vi "Create Suspected Pixels List.vi"(6 "IP Results":T1, 9 "tolerance":i32, 10 "Y Points":i16[](array[numeric]), 11 "X Points":i16[](array[numeric])) -> (1 "SuspPixelsIndex":u32[](array[numeric]), 2 "SuspPixelsY":u32[](array[numeric]), 3 "SuspPixelsX":u32[](array[numeric]))   [LabVIEW 2015]
uses:
  IP results.ctl
panel:
  out "Intensity Graph":u8[][](graph)
  out "Amount":i32
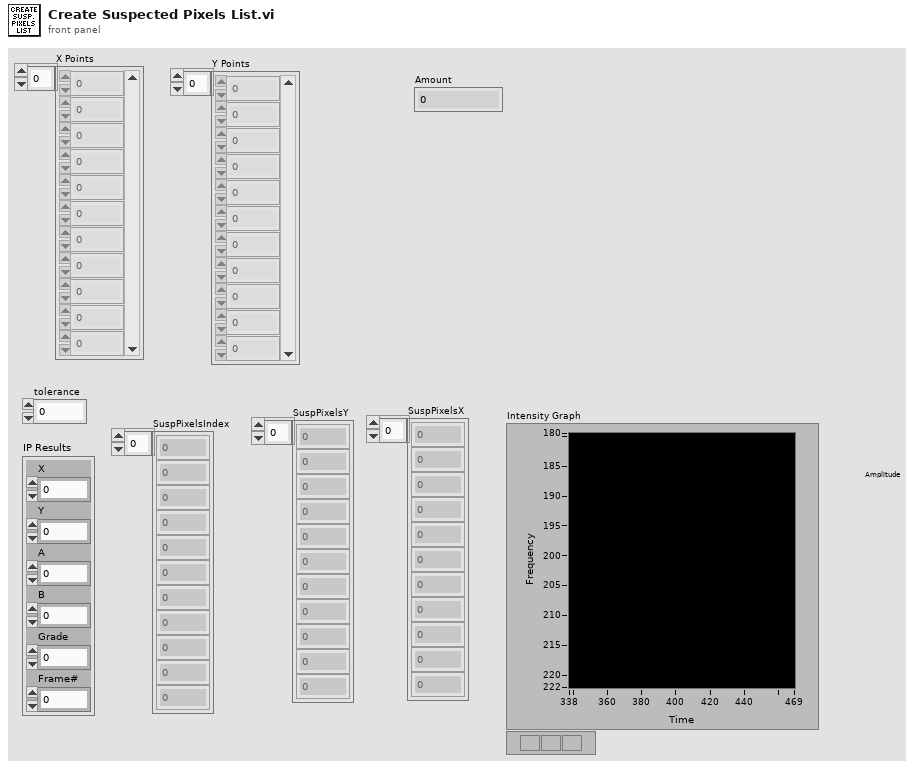
[diagram p1: front panel]
types:
  T1 = typedef "IP results.ctl" = cluster{"X":u16, "Y":u16, "A":dbl, "B":dbl, "Grade":u16, "Frame#":u16}
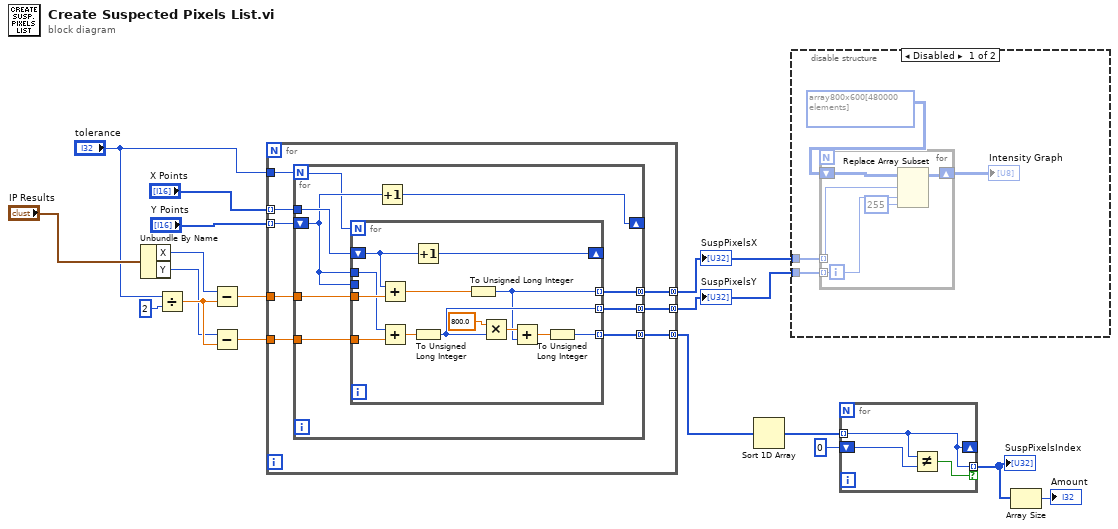
[diagram p0: block diagram]
diagram:
  n1 = Unbundle By Name("IP Results") -> ("X"=w9:u16, "Y"=w11:u16)
  n2 = Divide(x="tolerance", y=2) -> (x/y=w13:dbl)
  n3 = Subtract(x=w9, y=w13) -> (x-y=w10:dbl)
  n4 = Subtract(x=w11, y=w13) -> (x-y=w12:dbl)
  n5 = for {
    tunnel: "X Points" -> [w25] mode=indexing
    tunnel: "Y Points" -> [w24] mode=indexing
    tunnel: w10 -> [w23]
    tunnel: w12 -> [w22]
    tunnel: [w21] -> w1 mode=concatenating
    tunnel: [w20] -> w2 mode=concatenating
    tunnel: [w19] -> w15 mode=concatenating
    tunnel: "tolerance" -> [w18]
    n6 = for {
      N: w18 -> [w26]
      tunnel: w25 -> [w33]
      tunnel: w23 -> [w34]
      tunnel: w22 -> [w28]
      shift-right: [w32] -> _
      shift-left: w24 -> [w31]
      tunnel: [w30] -> w21 mode=concatenating
      tunnel: [w29] -> w20 mode=concatenating
      tunnel: [w27] -> w19 mode=concatenating
      n7 = for {
        N: w26 -> [_]
        tunnel: w34 -> [w47]
        tunnel: w31 -> [_]
        shift-right: [w46] -> _
        shift-left: w33 -> [w45]
        tunnel: [w37] -> w30 mode=indexing
        tunnel: [w39] -> w29 mode=indexing
        tunnel: w31 -> [w43]
        tunnel: w28 -> [w42]
        tunnel: [w35] -> w27 mode=indexing
        n8 = Add(x=w45, y=w47) -> (x+y=w44:dbl)
        n9 = Add(x=w43, y=w42) -> (x+y=w41:dbl)
        n10 = Increment(x=w45) -> (x+1=w46:i16)
        n11 = To Unsigned Long Integer(number=w41) -> (unsigned 32bit integer=w39:u32)
        n12 = To Unsigned Long Integer(number=w44) -> (unsigned 32bit integer=w37:u32)
        n13 = Multiply(x=800.0, y=w39) -> (x*y=w38:dbl)
        n14 = Add(x=w38, y=w37) -> (x+y=w36:dbl)
        n15 = To Unsigned Long Integer(number=w36) -> (unsigned 32bit integer=w35:u32)
      }
      n16 = Increment(x=w31) -> (x+1=w32:i16)
    }
  }
  "SuspPixelsY" <- w2
  "SuspPixelsX" <- w1
  n17 = Sort 1D Array(array=w15) -> (sorted array=w16:u32[])
  n18 = disable-structure shown="Disabled" {
    disable-tunnel: w2 -> [w50 _]
    disable-tunnel: w1 -> [w49 _]
    frame Disabled {
      n19 = for {
        shift-right: [w54] -> w48
        shift-left: u8[][] array800x600[480000 elements] -> [w56]
        tunnel: w50 -> [w52] mode=indexing
        tunnel: w49 -> [w53] mode=indexing
        n20 = Replace Array Subset(array=w56, new element=u8 255 ("new element/subarray"), index (row)=w53, index (col)=w52) -> (w54:u8[][])
      }
      "Intensity Graph" <- w48
    }
    frame Enabled {
    }
  }
  n21 = for {
    tunnel: w16 -> [w58] mode=indexing
    shift-right: [w58] -> _
    shift-left: u32 0 -> [w59]
    tunnel: [w58] -> w4 mode=indexing if=w57
    n22 = Not Equal?(x=w58, y=w59) -> (x != y?=w57:bool)
  }
  "SuspPixelsIndex" <- w4
  n23 = Array Size(array=w4) -> (size(s)=→"Amount":i32)
